vi "DAQ_testing.vi"() -> ()   [LabVIEW 2020]
uses:
  <vilib>/DAQmx/read.llb/DAQmx Read (Analog 1D Wfm NChan NSamp).vi
  <vilib>/Analysis/baseanly.llb/Mean (DBL).vi
  <vilib>/DAQmx/create/channels.llb/DAQmx Create Channel (AI-Voltage-Basic).vi
  <vilib>/DAQmx/configure/timing.llb/DAQmx Timing (Sample Clock).vi
  <vilib>/DAQmx/miscellaneous.llb/DAQmx Fill In Error Info.vi
  <vilib>/Analysis/NI_AALBase.lvlib
panel:
  out "Coupling":dbl format="%#_g%%"
  out "Degrees":dbl[](array[numeric])
  out "Volts":dbl[](array[numeric])
  out "Sensor Sampling":waveform(dbl)[](graph)
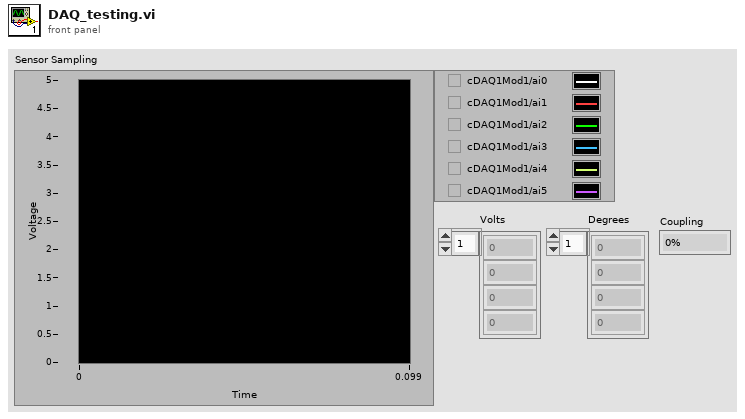
[diagram p1: front panel]
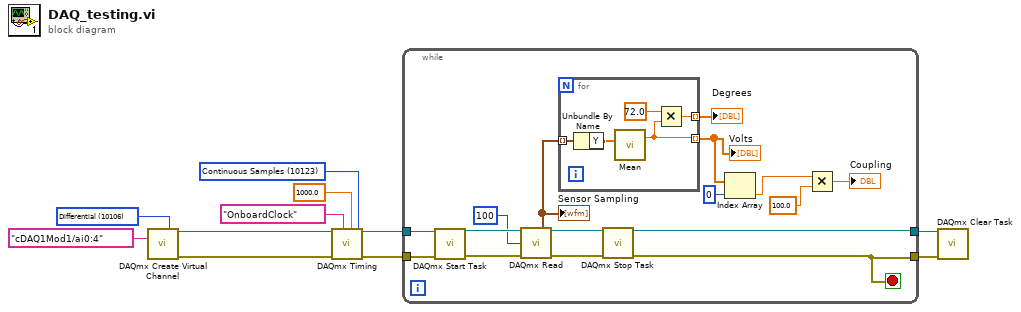
[diagram p0: block diagram]
diagram:
  w10 = 10106 items=["Default"=-1, "RSE"=10083, "NRSE"=10078, "Differential"=10106, "Pseudodifferential"=12529] ("input terminal configuration")
  w11 = 10123 items=["Finite Samples"=10178, "Continuous Samples"=10123, "Hardware Timed Single Point"=12522] ("sample mode")
  n1 = call-poly <vilib>:"DAQmx Create Virtual Channel.vi"("input terminal configuration"=w10, "physical channels"=tag "cDAQ1Mod1/ai0:4" ("DAQmx Physical Channel")) -> ("task out"=w6:refnum<k21>, "error out"=w7:errorcluster)  [unwired: 12 in]
  n2 = call-poly <vilib>:"DAQmx Timing.vi"("task/channels in"=w6, "sample mode"=w11, "rate"=1000.0 ("sample rate"), "source"=tag "OnboardClock", "error in"=w7) -> ("task out"=w4:refnum<k21>, "error out"=w3:errorcluster)  [unwired: 9 in]
  n3 = while {
    tunnel: w4 -> [w22]
    tunnel: w3 -> [w21]
    tunnel: [w20] -> w2
    tunnel: [w12] -> w1
    stop <- w12 stop-if-true
    n4 = call <vilib>:"DAQmx Start Task.vi"("task/channels in"=w22, "error in"=w21) -> ("task out"=w24:refnum<k21>, "error out"=w25:errorcluster)  [unwired: 12 in]
    n5 = call-poly <vilib>:"DAQmx Read.vi"("task/channels in"=w24, "number of samples per channel"=100 ("n samples/channel"), "error in"=w25) -> ("data"=w19:waveform(dbl)[], "task out"=w26:refnum<k21>, "error out"=w27:errorcluster)  [unwired: 10 in]
    "Sensor Sampling" <- w19
    n6 = for {
      tunnel: w19 -> [w32] mode=indexing
      tunnel: [w30] -> w17 mode=indexing
      tunnel: [w28] -> w18 mode=indexing
      n7 = Unbundle By Name(w32) -> ("Y"=w31:dbl[])
      n8 = call-poly <vilib>:"Mean.vi"("X"=w31) -> ("mean"=w30:dbl)  [unwired: 1 out]
      n9 = Multiply(x=72.0, y=w30) -> (x*y=w28:dbl)
    }
    "Volts" <- w17
    "Degrees" <- w18
    n10 = call <vilib>:"DAQmx Stop Task.vi"("task/channels in"=w26, "error in"=w27) -> ("task out"=w20:refnum<k21>, "error out"=w12:errorcluster)  [unwired: 12 in]
    n11 = Index Array(array=w17, index=0) -> (element=w14:dbl)
    n12 = Multiply(x=w14, y=100.0) -> (x*y=→"Coupling":dbl)
  }
  n13 = call <vilib>:"DAQmx Clear Task.vi"("task in"=w2, "error in"=w1) -> ()  [unwired: 13 in, 1 out]
